vi "Copy_Files.vi"(8 "error in (no error)":errorcluster, 11 "Build in":refnum<class "AB_EXE.lvclass">) -> (0 "error out":errorcluster, 3 "Build out":refnum<class "AB_EXE.lvclass">)   [LabVIEW 2020, in "AB_EXE.lvclass"]
uses:
  <vilib>/AppBuilder/AB_Classes/EXE/AB_EXE.lvclass
  e:/builds/penguin/labview/branches/2020/dev/dist/vi.lib/AppBuilder/AB_Classes/Build/AB_Build.lvclass
  <vilib>/AppBuilder/AB_Classes/Application/AB_Application.lvclass
  <vilib>/AppBuilder/AB_Classes/Destination/AB_Destination.lvclass
  <vilib>/AppBuilder/AB_Classes/Build/AB_Build.lvclass
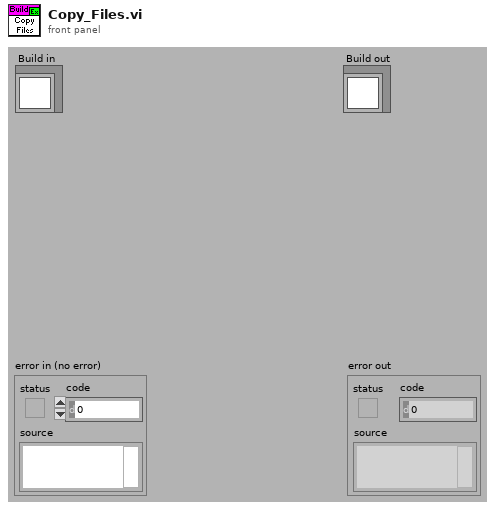
[diagram p1: front panel]
types:
  T1 = typedef "AB_Build.ctl" = cluster{"buildSpecName":string, "buildSpecDescription":string, "destinations":refnum<class "AB_Destination.lvclass">[], "exclusionOption":T2, "defaultLanguage":string, "supportedLanguages":string[], "excludedDirectories":path[], "buildContext":refnum<vi>, "buildObject":T3, "preview":bool, "programatic":bool, "progressBarEvents":T4, "userLog_Path":path, "preActionID":string, "preAction_Path":path, "postActionID":string, "postAction_Path":path, "eng_checkForBrokenVIs?":bool, "eng_verboseLinkerErrors?":bool, "localDest_Path":path, "targetDest_Path":path, "removeVIObject":u16, "cache":refnum<class "PreviewCache.lvclass">, "use cache":bool, "previewCache_ID":string, "buildCache_ID":string, "eng_TempLocalDest_Path":path, "eng_collectDependencies?":bool, "versionInfo":cluster{"buildVersion":cluster{"major":u16, "minor":u16, "patch":u16, "build":u16}, "autoIncrement":bool}, "eng_enableVIChecksums":bool}
  T2 = typedef "AB_Exclusion_Option.ctl" = cluster{"typedefs":bool, "polymorphicVIs":bool, "unusedLibraryItems":bool, "modifyLibraryFile":bool, "edit-timeDependencies":bool, "inlineVIs":bool, "dependent PPLs":bool, "dependent DLLs":bool}
  T3 = typedef "ItemRef.ctl" = u64
  T4 = typedef "provcom_ProgressBar_Events.ctl" = cluster{"newJob":refnum<user-event>, "newItem":refnum<user-event>, "errorMsg":T5, "cancel":refnum<user-event>}
  T5 = typedef "mxLvBuildError.ctl" = refnum<user-event>
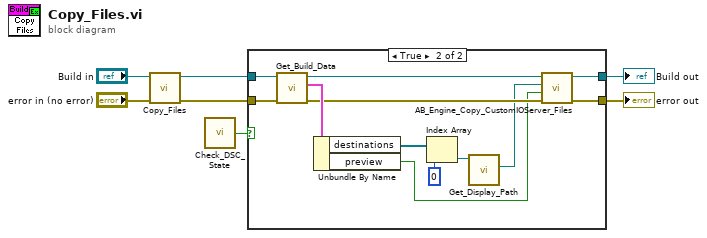
[diagram p0: block diagram]
diagram:
  n1 = call-parent "Copy_Files.vi"("error in (no error)"="error in (no error)", "Build in"="Build in") -> ("error out"=w2:errorcluster, "Build out"=w1:refnum<class "AB_EXE.lvclass">)  [unwired: 8 out]
  n2 = call <vilib>:"Check_DSC_State.vi"() -> ("active"=w3:bool)  [unwired: 1 out]
  n3 = case shown="True" w3 {
    tunnel: w2 -> [w8 w20]
    tunnel: w1 -> [w9 w17]
    tunnel: [w9 w16] -> w5
    tunnel: [w8 w15] -> w4
    frame False {
    }
    frame True {
      n4 = call <vilib>:"Get_Build_Data.vi"("error in (no error)"=w20, "Class in"=w17) -> ("error out"=w19:errorcluster, "data"=w21:T1, "Class out"=w18:refnum<class "AB_EXE.lvclass">)  [unwired: 7 out]
      n5 = Unbundle By Name(w21) -> ("destinations"=w12:refnum<class "AB_Destination.lvclass">[], "preview"=w10:bool)
      n6 = Index Array(array=w12, index=0) -> (element=w13:refnum<class "AB_Destination.lvclass">)
      n7 = call-dynamic "Get_Display_Path.vi"("AB_Destination in"=w13) -> ("displayPath"=w11:path)  [unwired: 1 in, 9 out]
      n8 = call <vilib>:"AB_Engine_Copy_CustomIOServer_Files.vi"("error in (no error)"=w19, "Preview?"=w10, "OutputDirectory"=w11, "Build in"=w18) -> ("error out"=w15:errorcluster, "Build out"=w16:refnum<class "AB_EXE.lvclass">)  [unwired: 6 out]
    }
  }
  "error out" <- w4
  "Build out" <- w5
